vi "To Variant.vi"(8 "Error In":errorcluster, 11 "TD Flt":refnum<class "Flt.lvclass">) -> (0 "Error Out":errorcluster, 2 "Variant":variant)   [LabVIEW 2017, in "Tree API.lvlib" / "Flt.lvclass"]
doc: "Dynamic dispatch interface for conversion of Tree Data classes to variant LV data."
uses:
  Flt.lvclass
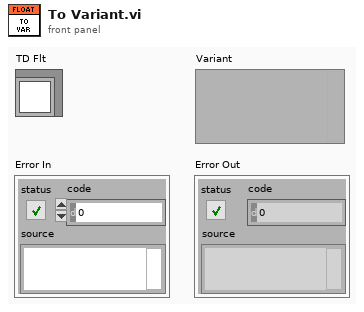
[diagram p1: front panel]
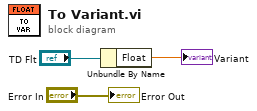
[diagram p0: block diagram]
diagram:
  n1 = Unbundle By Name("TD Flt") -> ("Float"=→"Variant":dbl)
  "Error Out" <- "Error In"
